vi "hse-application_GetUserDefinedPath.vi"(8 "error in":errorcluster, 11 "Name":string) -> (0 "error out":errorcluster, 3 "Path":path)   [LabVIEW 2022 SP3, in "hse-application.lvclass"]
doc: "returns the user defined path with the specified name\n\n____\nHAMPEL SOFTWARE ENGINEERING v3.8.0 (2023-12-18 14:41)"
uses:
  hse-application.lvclass
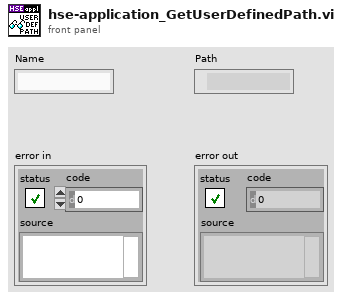
[diagram p1: front panel]
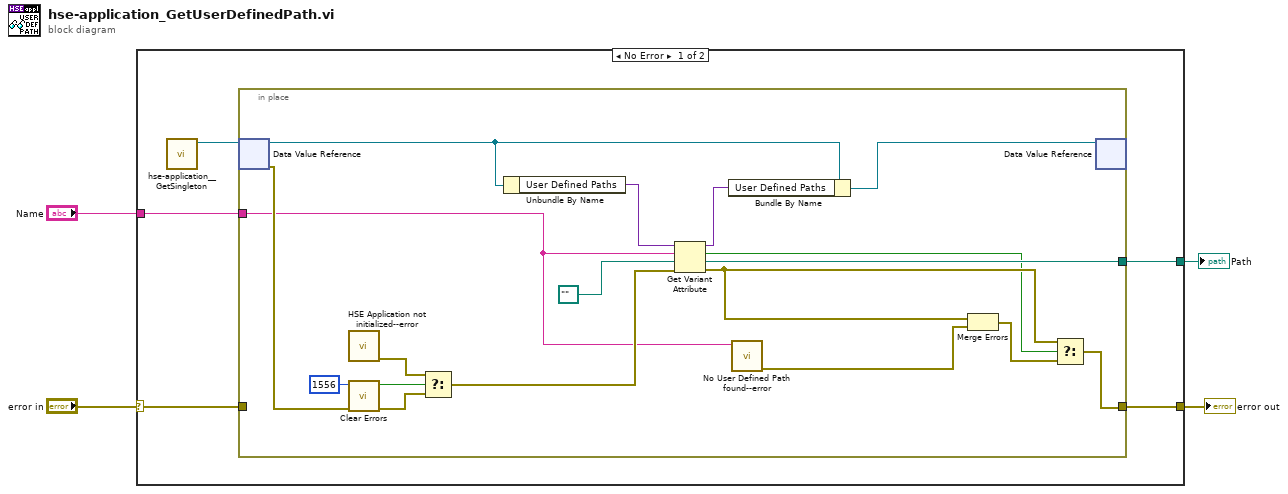
[diagram p0: block diagram]
diagram:
  n1 = case shown="No Error" "error in" {
    selector: "error in" -> [w9 w28]
    tunnel: [w8 w28] -> w3
    tunnel: "Name" -> [w7 _]
    tunnel: [w6 _] -> w1
    frame No Error {
      n2 = call "hse-application__GetSingleton.vi"() -> ("ApplicationClass DVR"=w5:refnum<data-value>)  [unwired: 10 in, 1 out]
      n3 = in-place "In Place Element Structure" {
        in-place-border: w9 -> [_]
        in-place-border: [w26] -> w8
        in-place-border: w7 -> [w10]
        in-place-border: [w17] -> w6
        n4 = in-place-dvr #1(w5) -> (w15:refnum<class "hse-application.lvclass">, w22:errorcluster)
        n5 = call "HSE Application not initialized--error.vi"() -> ("error out"=w24:errorcluster)  [unwired: 11 in]
        n6 = call <vilib>:"Clear Errors.vi"("error in (no error)"=w22, "specific error code to clear (0: all)"=1556) -> ("error out"=w23:errorcluster, "specific error cleared?"=w12:bool)  [unwired: 4 in]
        n7 = Select(t=w24, s=w12, f=w23) -> (s? t:f=w21:errorcluster)
        n8 = Unbundle By Name(w15) -> ("User Defined Paths"=w20:variant)
        n9 = Get Variant Attribute(Variant=w20, name=w10, default value (empty Variant)=path "", error in=w21) -> (duplicate Variant=w19:variant, found=w16:bool, value=w17:path, error out=w25:errorcluster)
        n10 = Bundle By Name(cluster=w15, "User Defined Paths"=w19) -> (w14:refnum<class "hse-application.lvclass">)
        n11 = call "No User Defined Path found--error.vi"("Additional Info"=w10) -> ("error out"=w11:errorcluster)  [unwired: 10 in]
        n12 = Merge Errors(w25, w11) -> (w27:errorcluster)
        n13 = Select(t=w25, s=w16, f=w27) -> (s? t:f=w26:errorcluster)
        n14 = in-place-dvr #1(w14) -> ()  [unwired: 2 out]
      }
    }
    frame Error {
    }
  }
  "error out" <- w3
  "Path" <- w1
